vi "AuMT8852B Loopback Test.vi"(7 "Settings":T1={"Pattern"=enum."PRBS-9", "Hop type"=enum."Fixed", "TX channel"=0, "RX channel"=39, "Packet type"=enum."DH1", "Data length"=27, "Dirty table"=enum."Dirty table disabled", "Dirty table index"=0, "Dirty table window"=1, "Number of packets"=0, "Whitening"=enum."Whitening disabled"}, 8 "error in (no error)":errorcluster, 11 "VISA session":refnum<visa-resource-name>) -> (0 "error out":errorcluster, 2 "error code":i32, 3 "VISA session out":refnum<visa-resource-name>)   [LabVIEW 2017]
doc: "Anritsu MT8852B Bluetooth Tester\n\nPerforms a single loopback test control sequence. The EUT must be connected and in test mode.\n\nUsage Notes: EUT must be in Test Mode before using this VI. Use Put EUT in Test Mode.vi. If Dirty Table is enabled, use Copy Dirty Table to Loopback Test.vi before using this VI.\n\nINPUTS\nSettings - parameters of the loopback test."
panel:
  # "Usage Notes: EUT must be in Test Mode before using this VI. Use Put EUT in Test Mode.vi.\nIf Dirty Table is enabled, use Copy Dirty Table to Loopback Test.vi before using this VI."
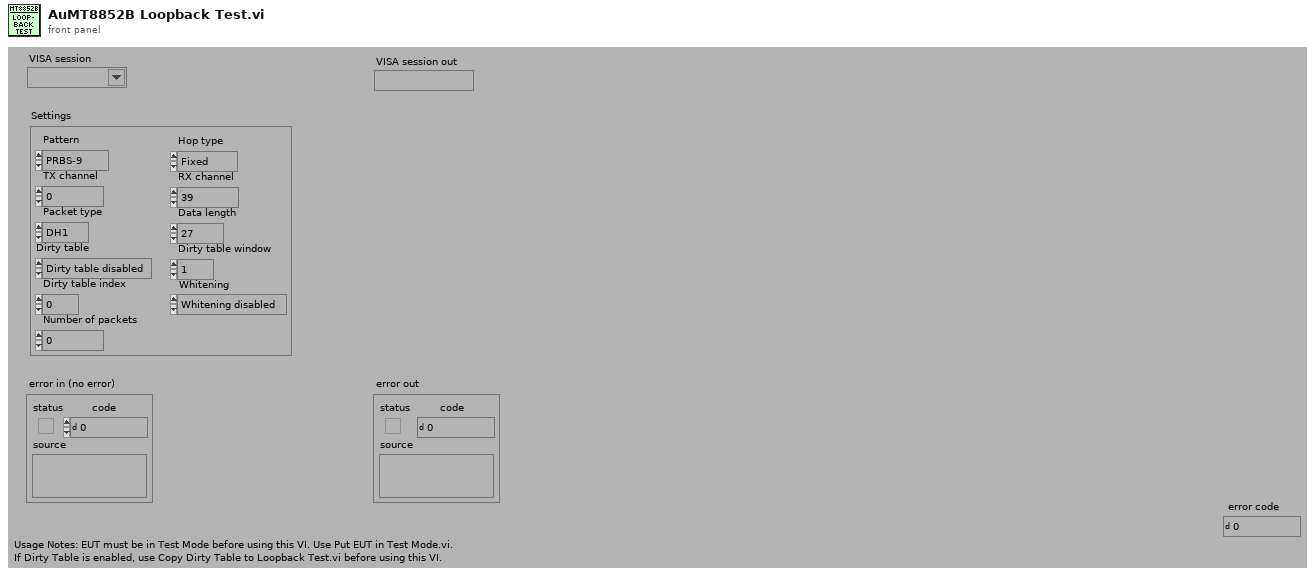
[diagram p1: front panel]
types:
  T1 = cluster{"Pattern":enum16{"10101010", "11110000", "PRBS-9"}, "Hop type":enum16{"Fixed", "Standard"}, "TX channel":i32, "RX channel":i32, "Packet type":enum16{"DH5", "DH3", "DH1"}, "Data length":i32, "Dirty table":enum16{"Dirty table disabled", "Dirty table enabled"}, "Dirty table index":i32, "Dirty table window":i32, "Number of packets":i32, "Whitening":enum16{"Whitening disabled", "Whitening enabled"}}
  T2 = enum16{"Simulate", "Range check", "Cache", "Query instrument status"}
  T3 = enum16{"Dirty table disabled", "Dirty table enabled"}
  T4 = enum16{"Whitening disabled", "Whitening enabled"}
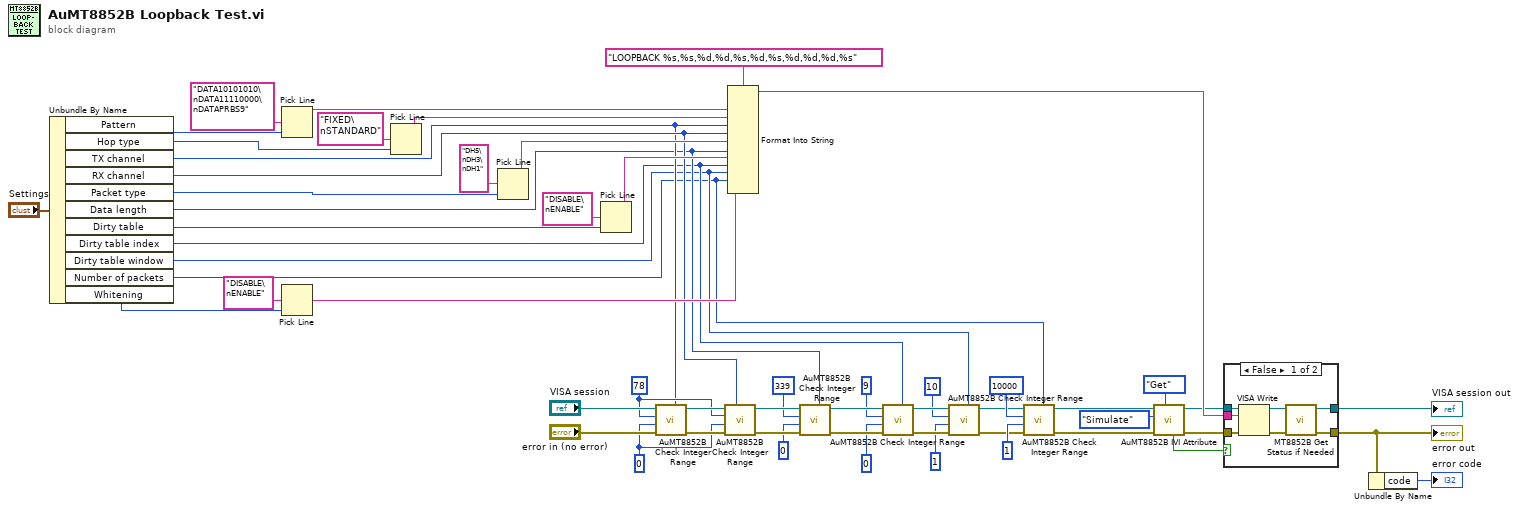
[diagram p0: block diagram]
diagram:
  w27 = 0 ("Lower limit (-1)")
  w28 = 78 ("Upper limit (1)")
  n1 = Unbundle By Name("Settings") -> ("Pattern"=w54:enum16{"10101010", "11110000", "PRBS-9"}, "Hop type"=w51:enum16{"Fixed", "Standard"}, "TX channel"=w25:i32, "RX channel"=w26:i32, "Packet type"=w49:enum16{"DH5", "DH3", "DH1"}, "Data length"=w22:i32, "Dirty table"=w48:T3, "Dirty table index"=w11:i32, "Dirty table window"=w10:i32, "Number of packets"=w9:i32, "Whitening"=w47:T4)
  n2 = Pick Line(multi-line string="DATA10101010\nDATA11110000\nDATAPRBS9", line index=w54) -> (output string=w44:string)  [unwired: 1 in]
  n3 = Pick Line(multi-line string="DISABLE\nENABLE", line index=w47) -> (output string=w39:string)  [unwired: 1 in]
  n4 = Pick Line(multi-line string="FIXED\nSTANDARD", line index=w51) -> (output string=w43:string)  [unwired: 1 in]
  n5 = Pick Line(multi-line string="DH5\nDH3\nDH1", line index=w49) -> (output string=w42:string)  [unwired: 1 in]
  n6 = Pick Line(multi-line string="DISABLE\nENABLE", line index=w48) -> (output string=w40:string)  [unwired: 1 in]
  n7 = call <instrlib>:"AuMT8852B Check Integer Range.vi"("Value (0)"=w25, "error in (no error)"="error in (no error)", "Lower limit (-1)"=w27, "Upper limit (1)"=w28, "VISA session"="VISA session") -> ("error out"=w29:errorcluster, "VISA session out"=w30:refnum<visa-resource-name>)  [unwired: 5 in]
  n8 = call <instrlib>:"AuMT8852B Check Integer Range.vi"("Set/Get (Set)"=w26, "error in (no error)"=w29, "Lower limit (-1)"=w27, "Upper limit (1)"=w28, "VISA session"=w30) -> ("error out"=w23:errorcluster, "VISA session out"=w24:refnum<visa-resource-name>)  [unwired: 5 in]
  n9 = Format Into String(format string="LOOPBACK %s,%s,%d,%d,%s,%d,%s,%d,%d,%d,%s" ("Format String"), w44, w43, w25, w26, w42, w22, w40, w11, w10, w9, w39) -> (resulting string=w38:string)  [unwired: 2 in, 1 out]
  n10 = call <instrlib>:"AuMT8852B Check Integer Range.vi"("Value (0)"=w22, "error in (no error)"=w23, "Lower limit (-1)"=0, "Upper limit (1)"=339, "VISA session"=w24) -> ("error out"=w12:errorcluster, "VISA session out"=w13:refnum<visa-resource-name>)  [unwired: 5 in]
  n11 = call <instrlib>:"AuMT8852B Check Integer Range.vi"("Value (0)"=w11, "error in (no error)"=w12, "Lower limit (-1)"=0, "Upper limit (1)"=9, "VISA session"=w13) -> ("error out"=w15:errorcluster, "VISA session out"=w14:refnum<visa-resource-name>)  [unwired: 5 in]
  n12 = call <instrlib>:"AuMT8852B Check Integer Range.vi"("Value (0)"=w10, "error in (no error)"=w15, "Lower limit (-1)"=1 ("Upper limit (1)"), "Upper limit (1)"=10, "VISA session"=w14) -> ("error out"=w17:errorcluster, "VISA session out"=w16:refnum<visa-resource-name>)  [unwired: 5 in]
  n13 = call <instrlib>:"AuMT8852B Check Integer Range.vi"("Value (0)"=w9, "error in (no error)"=w17, "Lower limit (-1)"=1, "Upper limit (1)"=10000, "VISA session"=w16) -> ("error out"=w7:errorcluster, "VISA session out"=w8:refnum<visa-resource-name>)  [unwired: 5 in]
  n14 = call <instrlib>:"AuMT8852B IVI Attribute.vi"("Set/Get (Set)"=enum16{"Set", "Get"}."Get", "error in (no error)"=w7, "Flag (Simulate)"=T2."Simulate", "VISA session"=w8) -> ("error out"=w37:errorcluster, "VISA session out"=w36:refnum<visa-resource-name>, "Value out"=w35:bool)  [unwired: 5 in]
  n15 = case shown="False" w35 {
    tunnel: [w63 w65] -> w56
    tunnel: [w62 w64] -> w5
    tunnel: w37 -> [w59 w64]
    tunnel: w36 -> [w58 w65]
    tunnel: w38 -> [w57 _]
    frame False {
      n16 = VISA Write(VISA resource name=w58, write buffer=w57, error in (no error)=w59) -> (VISA resource name out=w60:refnum<visa-resource-name>, error out=w61:errorcluster)  [unwired: 1 out]
      n17 = call <instrlib>:"MT8852B Get Status if Needed.vi"("error in (no error)"=w61, "VISA session"=w60) -> ("error out"=w62:errorcluster, "VISA session out"=w63:refnum<visa-resource-name>)  [unwired: 8 in]
    }
    frame True {
    }
  }
  "error out" <- w5
  "VISA session out" <- w56
  n18 = Unbundle By Name(w5) -> ("code"=→"error code":i32)
